vi "Actor Core.vi"(8 "error in":errorcluster, 11 "T Controller in":refnum<class "Mag Lab Temperature Controller.lvclass">) -> (0 "error out":errorcluster, 3 "Actor out":refnum<class "Actor.lvclass">)   [LabVIEW 2015, in "Mag Lab Temperature Controller.lvclass"]
doc: "(<B>Filename</B>: Actor Framework.lvlib:Actor.lvclass:Actor Core.vi)\n\nReceives messages to the actor, reacts to them, and initiates any error handling that may shut the actor down.\n\nDescendant classes may override this VI to append parallel tasks for the actor to complete while it handles messages. Overrides use the Call Parent Method node."
uses:
  Mag Lab Temperature Controller.lvclass
  <vilib>/ActorFramework/Actor/Actor.lvclass
  T controller parameters.ctl
  Instruments/Neocera/Neocera Set Point Aproach.ctl
  Mag Lab Root/Mag Lab Root.lvclass/Mag Lab Root.ctl
  <vilib>/ActorFramework/Actor/Actor.lvclass/Actor.ctl
  <vilib>/ActorFramework/Message Enqueuer/Message Enqueuer.lvclass/Message Enqueuer.ctl
  <vilib>/ActorFramework/Message Enqueuer/Init from Existing Queue.vi
  <vilib>/ActorFramework/Message Enqueuer/Enqueue.vi
  <vilib>/ActorFramework/Message Priority Queue/Priority Enqueue.vi
  Source/Source.lvclass
  <vilib>/ActorFramework/Message Enqueuer/Message Enqueuer.lvclass
  Mag Lab Root Messages/Close Front Panel Msg/Close Front Panel Msg.lvclass
  Mag Lab Root/Mag Lab Root.lvclass
  Mag Lab Error Handler/Mag Lab Error Handler.lvclass
panel:
  in  "Close":bool
  in  "Parameters":T1={"Record heater"=FALSE, "Record RAW"=FALSE, "Set point"=0.0, "Heater range"=0.0, "Approach"=enum."Instant", "Ramp rate, K/min"=0.0, "Record Channels"=["A"], "Settling time "=60.0, "Settling range"=0.1, "P"=0.0, "I"=0.0, "D"=0.0, "Temperature Control"=FALSE}
  # "Temperature Monitor"
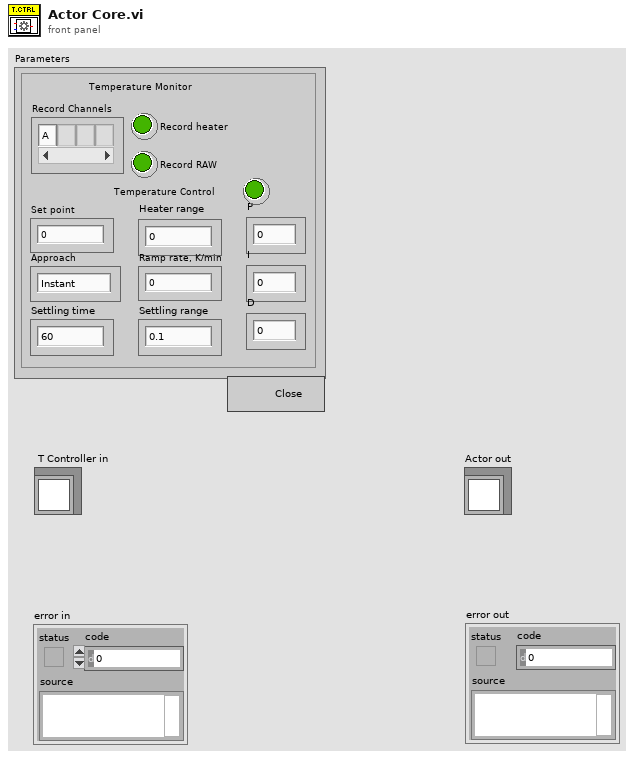
[diagram p1: front panel]
types:
  T1 = typedef "T controller parameters.ctl" = cluster{"Record heater":bool, "Record RAW":bool, "Set point":dbl, "Heater range":dbl, "Approach":T2, "Ramp rate, K/min":dbl, "Record Channels":string[], "Settling time ":dbl, "Settling range":dbl, "P":dbl, "I":dbl, "D":dbl, "Temperature Control":bool}
  T2 = typedef "Neocera Set Point Aproach.ctl" = enum16{"Instant", "Ramp"}
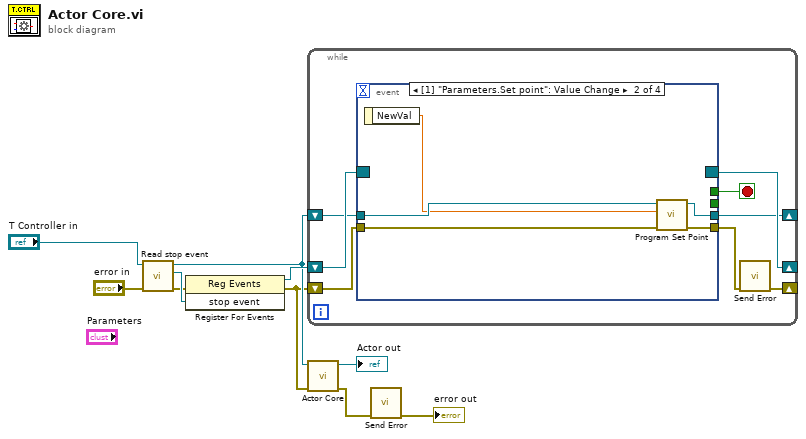
[diagram p0: block diagram]
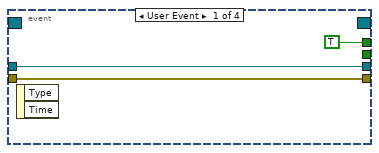
[diagram p2: hidden frame]
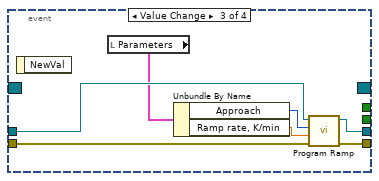
[diagram p3: hidden frame]
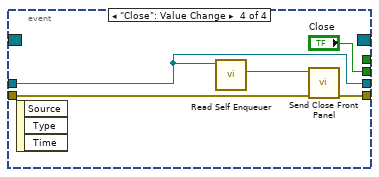
[diagram p4: hidden frame]
diagram:
  n1 = call "Read stop event.vi"("error in (no error)"="error in", "Mag Lab Root in"="T Controller in") -> ("error out"=w2:errorcluster, "stop event"=w7:refnum<user-event>, "Mag Lab Root out"=w5:refnum<class "Mag Lab Temperature Controller.lvclass">)  [unwired: 7 in]
  n2 = register-events(error in=w2, w7) -> (reference out=w6:refnum<event-registration>, error out=w1:errorcluster)  [unwired: 1 in]
  n3 = while {
    shift-right: [w17] -> _
    shift-left: w6 -> [w18]
    shift-right: [w14] -> _
    shift-left: w5 -> [w15]
    shift-right: [w12] -> _
    shift-left: w1 -> [w13]
    stop <- w16 stop-if-true
    n4 = event shown="[1] \"Parameters.Set point\": Value Change" {
      selector: w18 -> [_ _ _ _]
      dyn-events: [_ _ _ _] -> w17
      timeout: _ -> [_ _ _ _]
      tunnel: [TRUE _ _ _] -> w16
      tunnel: [_ _ _ "Close"] -> _
      tunnel: w15 -> [w20 w26 w33 w36]
      tunnel: [w20 w25 w32 w36] -> w14
      tunnel: w13 -> [w19 w24 w27 w34]
      tunnel: [w19 w23 w29 w35] -> w11
      event User Event {
        n5 = event-data() -> ()  [unwired: 1 in, 2 out]
      }
      event Value Change {
        n6 = event-data() -> ("NewVal"=w22:dbl)  [unwired: 1 in]
        n7 = call-dynamic "Program Set Point.vi"("error in (no error)"=w24, "Set Point"=w22, "Mag Lab Temperature Controller in"=w26) -> ("error out"=w23:errorcluster, "Mag Lab Temperature Controller out"=w25:refnum<class "Mag Lab Temperature Controller.lvclass">)  [unwired: 7 in]
      }
      event Value Change {
        n8 = event-data() -> ()  [unwired: 1 in, 1 out]
        n9 = local read "Parameters"() -> (w28:T1)
        n10 = Unbundle By Name(w28) -> ("Approach"=w31:T2, "Ramp rate, K/min"=w30:dbl)
        n11 = call-dynamic "Program Ramp.vi"("error in (no error)"=w27, "Ramp rate, K/min"=w30, "Approach"=w31, "Mag Lab Temperature Controller in"=w33) -> ("error out"=w29:errorcluster, "Mag Lab Temperature Controller out"=w32:refnum<class "Mag Lab Temperature Controller.lvclass">)  [unwired: 6 in]
      }
      event "Close": Value Change {
        n12 = event-data() -> ()  [unwired: 1 in, 3 out]
        n13 = call <vilib>:"Read Self Enqueuer.vi"("Actor"=w36) -> ("Self Enqueuer"=w37:refnum<class "Message Enqueuer.lvclass">)  [unwired: 10 in]
        n14 = call "Send Close Front Panel.vi"("error in (no error)"=w34, "Message Enqueuer"=w37) -> ("error out"=w35:errorcluster)  [unwired: 8 in, 1 out]
      }
    }
    n15 = call "Send Error.vi"("error in (no error)"=w11) -> ("error out"=w12:errorcluster)  [unwired: 9 in, 1 out]
  }
  n16 = call-parent "Actor Core.vi"("error in"=w1, "Mag Lab Measure Base in"=w5) -> ("error out"=w4:errorcluster, "Actor out"=→"Actor out":refnum<class "Actor.lvclass">)  [unwired: 8 in]
  n17 = call "Send Error.vi"("error in (no error)"=w4) -> ("error out"=→"error out":errorcluster)  [unwired: 9 in, 1 out]
